vi "Add Block Diagram Content.vi"(8 "error in (no error)":errorcluster, 9 "Term Refnum":refnum<vi>, 10 "ModuleLoop":T1, 11 "Input Signal in":refnum<class "Input Signal.lvclass">) -> (0 "error out":errorcluster, 3 "Input Signal out":refnum<class "Input Signal.lvclass">)   [LabVIEW 2015, in "Input Signal.lvclass"]
uses:
  Input Signal.lvclass
  Block Diagram/Block Diagram/Module.Refs.ctl
  <vilib>/Utility/miscctls.llb/LVPointTypeDef.ctl
  Block Diagram/Block Diagram/Block Diagram.lvclass
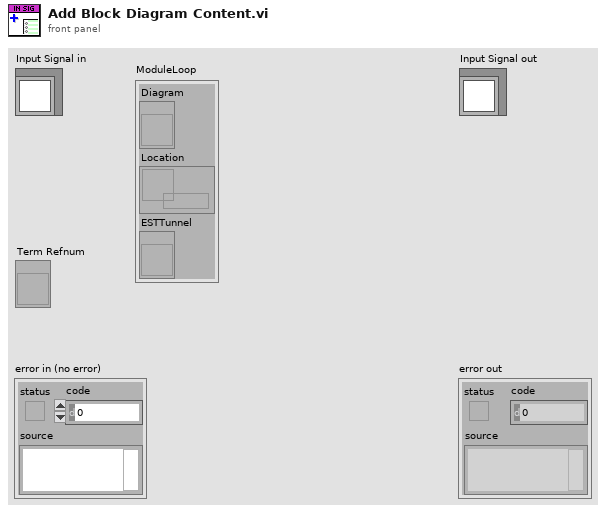
[diagram p1: front panel]
types:
  T1 = typedef "Block Diagram.lvclass/Module.Refs.ctl" = cluster{"Diagram":refnum<vi>, "Location":refnum<data-value>, "ESTTunnel":refnum<vi>}
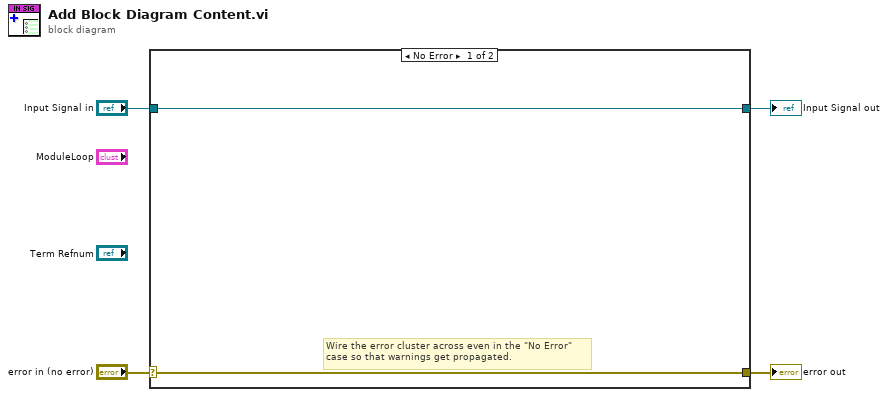
[diagram p0: block diagram]
diagram:
  n1 = case shown="No Error" "error in (no error)" {
    selector: "error in (no error)" -> [w5 w8]
    tunnel: [w5 w8] -> w3
    tunnel: [w6 w7] -> w1
    tunnel: "Input Signal in" -> [w6 w7]
    frame No Error {
      # "Wire the error cluster across even in the \"No Error\"\ncase so that warnings get propagated."
    }
    frame Error {
    }
  }
  "error out" <- w3
  "Input Signal out" <- w1
